vi "Run Pre-Compile.vi"(8 "Error In":errorcluster, 11 "Compiler In":refnum<class "Compiler.lvclass">) -> (0 "Error Out":errorcluster, 3 "Compiler Out":refnum<class "Compiler.lvclass">)   [LabVIEW 2018, in "Toolkit.lvlib" / "Compiler.lvclass"]
uses:
  Compiler.lvclass
  Hooks/Compile/Process/Process.lvclass
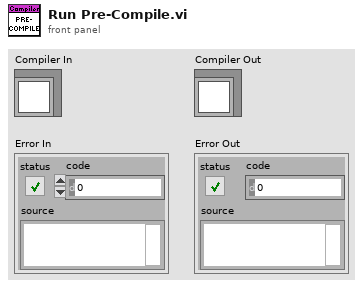
[diagram p1: front panel]
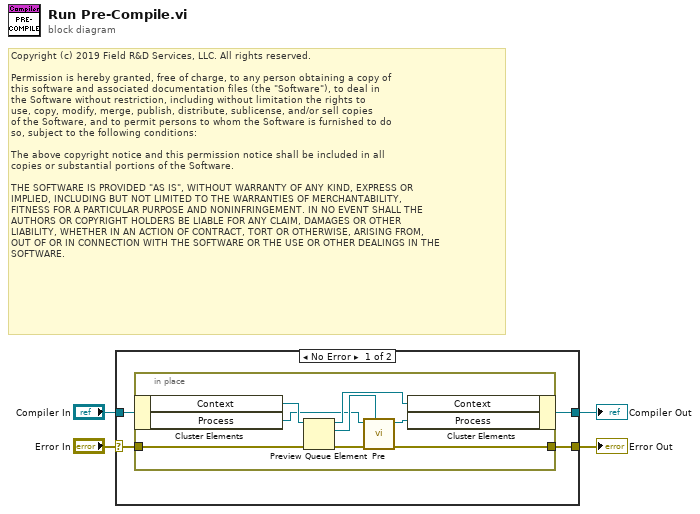
[diagram p0: block diagram]
diagram:
  # "Copyright (c) 2019 Field R&D Services, LLC. All rights reserved.\n\nPermission is hereby granted, free of charge, to any person obtaining a copy of\nthis software and associated documentation files (the \"Software\"), to deal in\nthe Software without restriction, including without limitation the rights to\nuse, copy, modify, merge, publish, distribute, sublicense, and/or sell copies\nof the Software, and to permit persons to whom the Software is furnished to do\nso, subject to the following conditions:\n\nThe above copyright notice and this permission notice shall be included in all\ncopies or substantial portions of the Software.\n\nTHE SOFTWARE IS PROVIDED \"AS IS\", WITHOUT WARRANTY OF ANY KIND, EXPRESS OR\nIMPLIED, INCLUDING BUT NOT LIMITED TO THE WARRANTIES OF MERCHANTABILITY,\nFITNESS FOR A PARTICULAR PURPOSE AND NONINFRINGEMENT. IN NO EVENT SHALL THE\nAUTHORS OR COPYRIGHT HOLDERS BE LIABLE FOR ANY CLAIM, DAMAGES OR OTHER\nLIABILITY, WHETHER IN AN ACTION OF CONTRACT, TORT OR OTHERWISE, ARISING FROM,\nOUT OF OR IN CONNECTION WITH THE SOFTWARE OR THE USE OR OTHER DEALINGS IN THE\nSOFTWARE."
  n1 = case shown="No Error" "Error In" {
    selector: "Error In" -> [w8 w17]
    tunnel: "Compiler In" -> [w5 w18]
    tunnel: [w7 w18] -> w2
    tunnel: [w6 w17] -> w1
    frame No Error {
      n2 = in-place {
        in-place-border: w8 -> [w13]
        in-place-border: [w16] -> w6
        n3 = in-place-cluster #1(w5) -> ("Context"=w15:refnum<queue>, "Process"=w10:refnum<class "Process.lvclass">)
        n4 = Preview Queue Element(queue=w15, error in (no error)=w13) -> (queue out=w14:refnum<queue>, element=w11:refnum<class "Datum.lvclass">, error out=w12:errorcluster)  [unwired: 1 in, 1 out]
        n5 = call-dynamic "Pre.vi"("Datum"=w11, "Error In"=w12, "Compile In"=w10) -> ("Error Out"=w16:errorcluster, "Compile Out"=w9:refnum<class "Process.lvclass">)  [unwired: 7 in]
        n6 = in-place-cluster #1("Context"=w14, "Process"=w9) -> (w7:refnum<class "Compiler.lvclass">)
      }
    }
    frame Error {
    }
  }
  "Compiler Out" <- w2
  "Error Out" <- w1
